vi "Test MQTT-3.1.3-1.vi"(8 "error in (no error)":errorcluster) -> (0 "error out":errorcluster)   [LabVIEW 2013]
uses:
  <vilib>/LabVIEW Open Source Project/MQTT Control Packets/Control Packets/CONNECT/ConnectFlags -- cluster.ctl
  <vilib>/addons/_JKI Toolkits/Caraya/classes/Assert/Assert Equal Value_Variant.vi
  <vilib>/LabVIEW Open Source Project/MQTT Control Packets/Control Packets/CONNECT/CONNECT.lvclass
  <vilib>/addons/_JKI Toolkits/Caraya/classes/Test/Test.lvclass
  <vilib>/addons/_JKI Toolkits/Caraya/classes/Assert/Assert.lvclass
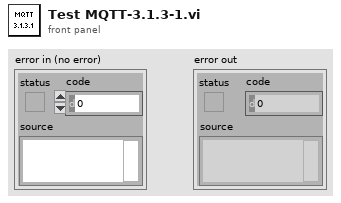
[diagram p1: front panel]
types:
  T1 = cluster{"Will Topic":string, "Will Message":string, "Username":string, "Password":string}
  T2 = typedef "MQTT_Control_Packets.lvlib/CONNECT.lvclass/ConnectFlags -- cluster.ctl" = cluster{"Reserved":bool, "Clean Session":bool, "Will Flag":bool, "Will QoS 1":bool, "Will QoS 2":bool, "Will Retain":bool, "Password Flag":bool, "User Name Flag":bool}
  T3 = typedef "MQTT_Control_Packets.lvlib/CONNECT.lvclass/ConnectPayload -- cluster.ctl" = cluster{"Will Topic":string, "Will Message":string, "Username":string, "Password":string}
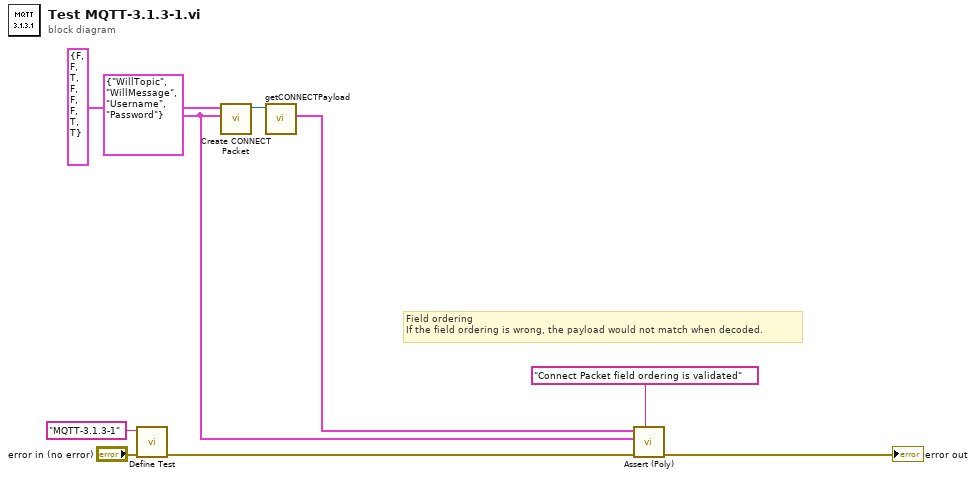
[diagram p0: block diagram]
diagram:
  w1 = T1 {"Will Topic"="WillTopic", "Will Message"="WillMessage", "Username"="Username", "Password"="Password"} ("Payload")
  # "Field ordering\nIf the field ordering is wrong, the payload would not match when decoded."
  n1 = call <vilib>:"Define Test.vi"("error in (no error)"="error in (no error)", "Label (VI Title)"="MQTT-3.1.3-1") -> ("error out"=w6:errorcluster)  [unwired: 9 in]
  n2 = call <vilib>:"Create CONNECT Packet.vi"("Payload"=w1, "Connect Flags"=T2 {"Reserved"=FALSE, "Clean Session"=FALSE, "Will Flag"=TRUE, "Will QoS 1"=FALSE, "Will QoS 2"=FALSE, "Will Retain"=FALSE, "Password Flag"=TRUE, "User Name Flag"=TRUE}) -> ("CONNECT"=w3:refnum<class "CONNECT.lvclass">)  [unwired: 7 in, 2 out]
  n3 = call <vilib>:"getCONNECTPayload.vi"("CONNECT in"=w3) -> ("Payload"=w2:T3)  [unwired: 9 in, 1 out]
  n4 = call-poly <vilib>:"Assert (Poly).vi"("Label"="Connect Packet field ordering is validated", "error in (no error)"=w6, "Y"=w1, "X"=w2) -> ("error out"=→"error out":errorcluster)  [unwired: 7 in]
